vi "Wellington1.vi"() -> ()   [LabVIEW 2009]
uses:
  <vilib>/NXT/Block Support/NXT_InputPort.ctl
  <vilib>/NXT/Block Support/NXT_ButtonSelector.ctl
  <vilib>/NXT/Subs/MotorOutput.ctl
  <vilib>/NXT/Dual Mode Library/Waits/Wait_Num.vi
  <vilib>/NXT/Dual Mode Library/Display/drawText.vi
  <vilib>/NXT/Dual Mode Library/Sensors/Light_On.vi
  <vilib>/NXT/Dual Mode Library/Sensors/Touch_Pressed.vi
  <vilib>/NXT/Dual Mode Library/Sensors/Sound_dB.vi
  <vilib>/NXT/Dual Mode Library/Sensors/Sonar_cm.vi
  <vilib>/NXT/Dual Mode Library/Sensors/readNXTButton.vi
  <vilib>/NXT/Subs/NXT_SteeringOutputPort.ctl
panel:
  out "Cor inicial":i16
  out "Verificacao":bool[](array[boolean])
  out "Toque":bool
  out "Visor":string
  out "Ruído":i16(slide) scale=0.0..100.0
  out "Luminosidade":i16
  out "Distância":i16
  out "Botao":bool
  # "O Mindstorms irá ficar no seguinte loop até que o botão central seja precionado:\nAciona os motores B e C para frente.\nMostrará os valores dos sensores na tela.\nCaso seja detectado: uma distância menor que 50cm, ou um ruído maior que 70dB, ou o sensor de toque seja precionado ou haja uma mudança de cor. O Mindstorms irá executar a seguinte rotina:\nIrá desligar os motores B e C.\nIrá ligar os motores B e C para trás e dará cinco voltas.\nSelecionará aleatoriamente um lado (direita/esquerda).\nEmitirá um som \"äleatório\".\nVirará 180 graus para o lado escolhido.\nE voltará ao loop."
  # "Configuração:\nOUT_A: GARRA\nOUT_B: RODA DA ESQUERDA\nOUT_C: RODA DA DIREITA\nIN_1: SENSOR DE TOQUE\nIN_2: SENSOR SONORO\nIN_3: SENSOR LUMINOSO\nIN_4: SENSOR ULTRA-SOM"
  # "1 - Distância menor que 50cm\n2 - Mudança de cor detectada\n3 - Ruído maior que 70dB\n4 - Toque precionado"
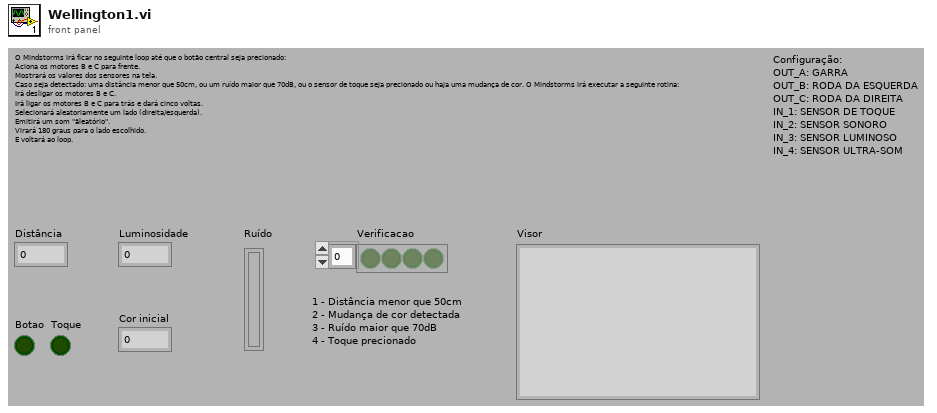
[diagram p1: front panel]
types:
  T1 = typedef "MotorOutput.ctl" = u8
  T2 = typedef "NXT_InputPort.ctl" = u8
  T3 = typedef "LVHSConnector.ctl" = cluster{"error":errorcluster, "address":string, "NXT #":i32, "Show Error":bool, "Connection":u16}
  T4 = typedef "NXT_SteeringOutputPort.ctl" = u16
  T5 = typedef "NXT_ButtonSelector.ctl" = u16
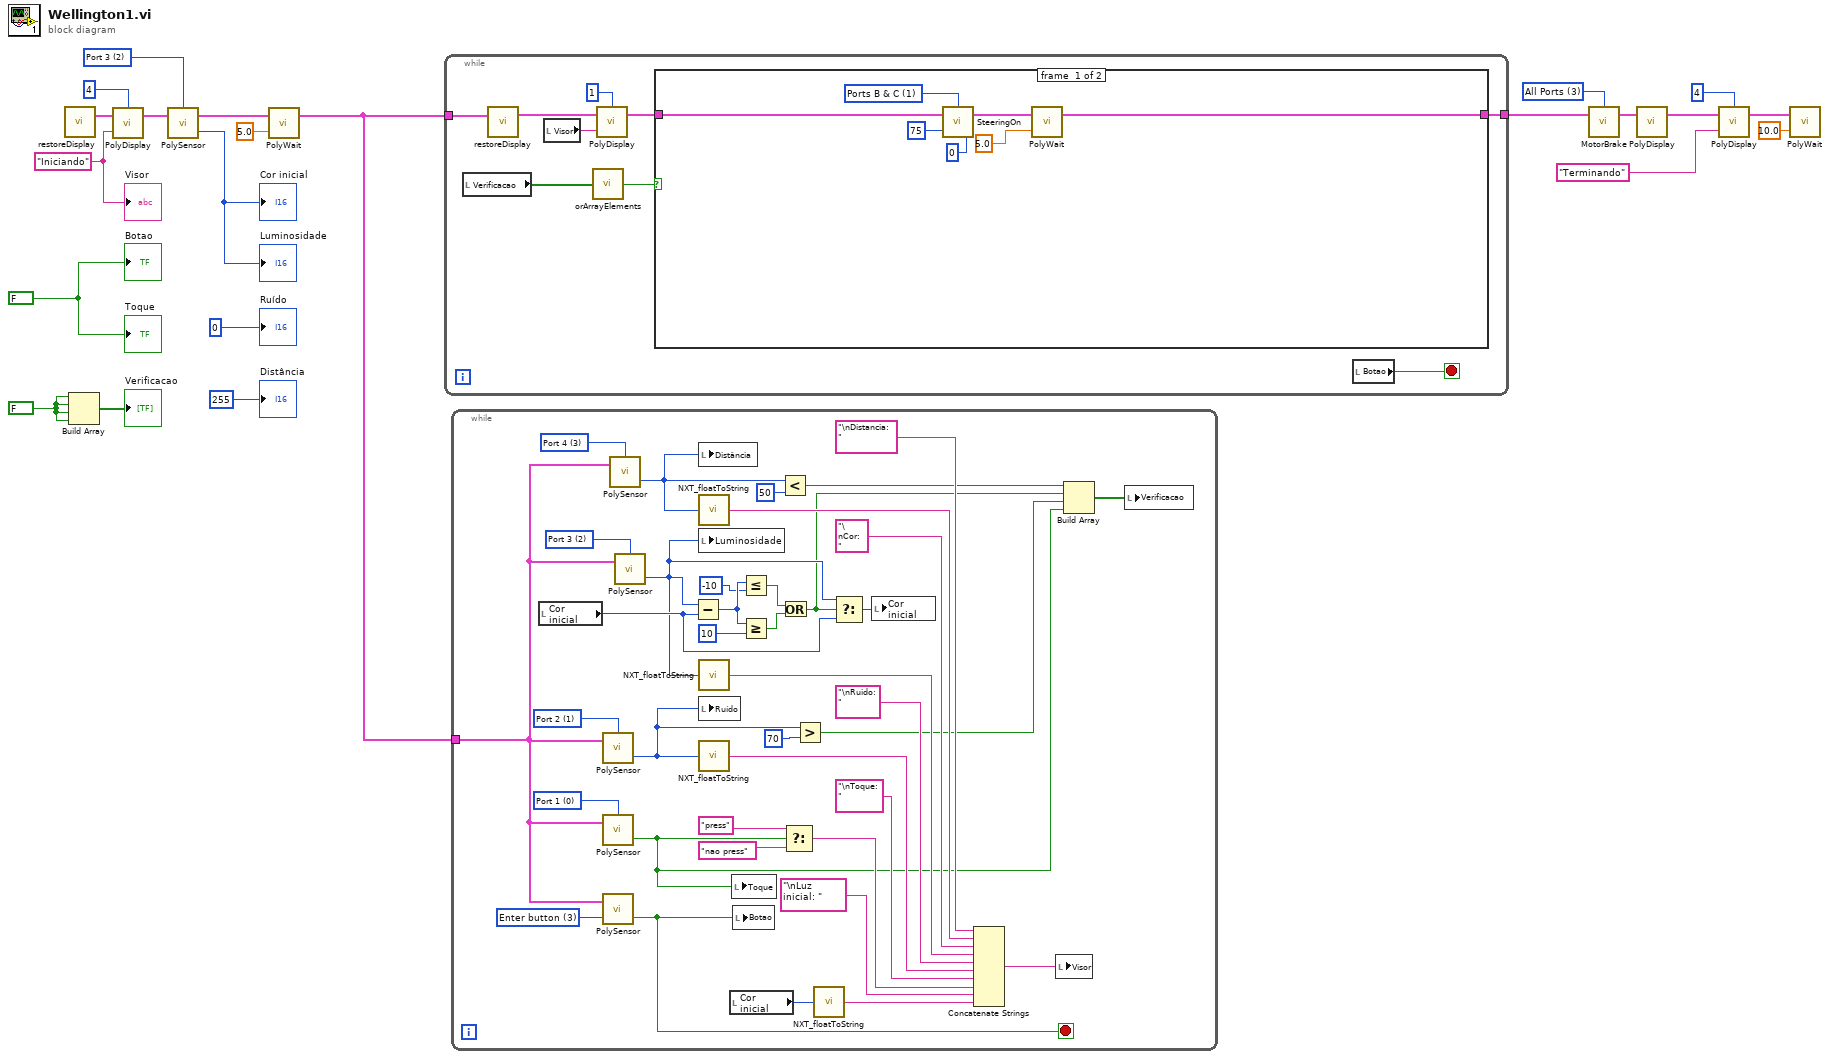
[diagram p0: block diagram]
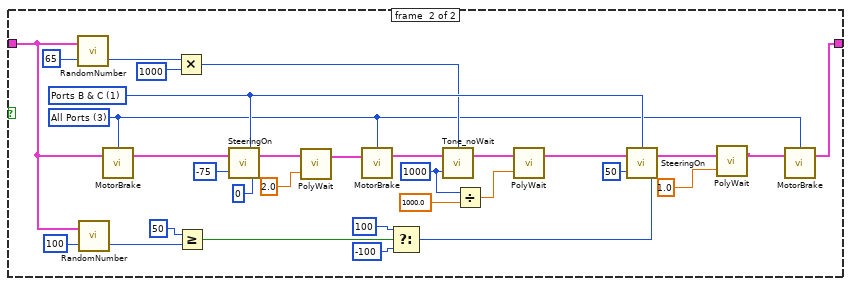
[diagram p2: hidden frame]
diagram:
  w3 = FALSE
  w14 = T1 3 items=["Port A", "Port B", "Port C", "All Ports"] ("Output Port (All Ports)")
  w10 = T2 2 items=["Port 1", "Port 2", "Port 3", "Port 4"] ("Input Port")
  w21 = "Iniciando"
  w20 = FALSE
  n1 = call <vilib>:"restoreDisplay.vi"() -> ("NXT"=w15:T3)  [unwired: 4 in]
  n2 = Build Array(w3, w3, w3, w3) -> (→"Verificacao":bool[])
  n3 = call-poly <vilib>:"PolyDisplay.vi"("Text"=w21, "NXT"=w15, "Line"=i16 4) -> ("NXT"=w7:T3)  [unwired: 1 in]
  n4 = call-poly <vilib>:"PolySensor.vi"("NXT"=w7, "Port (Port 3)"=w10) -> ("Scaled Value"=→"Luminosidade" →"Cor inicial":i16, "NXT"=w8:T3)  [unwired: 1 in]
  n5 = call-poly <vilib>:"PolyWait.vi"("Time (1 sec)"=sgl 5.0, "NXT"=w8) -> ("NXT"=w2:T3)  [unwired: 2 in]
  n6 = while {
    tunnel: w2 -> [w27]
    tunnel: [w23] -> w5
    stop <- w31 stop-if-true
    n7 = local read "Verificacao"() -> (w26:bool[])
    n8 = call <vilib>:"restoreDisplay.vi"("NXT"=w27) -> ("NXT"=w30:T3)  [unwired: 3 in]
    n9 = local read "Visor"() -> (w28:string)
    n10 = call <vilib>:"orArrayElements.vi"("Boolean Array"=w26) -> ("Logical OR"=w24:bool)
    n11 = call-poly <vilib>:"PolyDisplay.vi"("Text"=w28, "NXT"=w30, "Line"=i16 1) -> ("NXT"=w25:T3)  [unwired: 1 in]
    n12 = case shown="False" w24 {
      tunnel: w25 -> [w35 w66]
      tunnel: [w32 w41] -> w23
      frame #0 {
        w36 = T4 1 items=["Ports A & B", "Ports B & C", "Ports A & C"] ("Output Port")
        n13 = call <vilib>:"SteeringOn.vi"("Power (75)"=75, "Steering (100)"=0, "NXT"=w35, "Output Ports"=w36) -> ("NXT"=w34:T3)
        n14 = call-poly <vilib>:"PolyWait.vi"("Time (1 sec)"=sgl 5.0, "NXT"=w34) -> ("NXT"=w32:T3)  [unwired: 2 in]
      }
      frame #1 {
        w50 = u16 1000
        w48 = T1 3 items=["Port A", "Port B", "Port C", "All Ports"] ("Output Port (All Ports)")
        w65 = T4 1 items=["Ports A & B", "Ports B & C", "Ports A & C"] ("Output Port")
        n15 = call <vilib>:"RandomNumber.vi"("Max Value"=i16 65, "NXT"=w66) -> ("Random Number"=w61:u16)  [unwired: 1 in, 1 out]
        n16 = call <vilib>:"RandomNumber.vi"("Max Value"=i16 100, "NXT"=w66) -> ("Random Number"=w57:u16)  [unwired: 1 in, 1 out]
        n17 = call <vilib>:"MotorBrake.vi"("NXT"=w66, "Port (All Ports)"=w48) -> ("NXT"=w40:T3)  [unwired: 2 in]
        n18 = Multiply(x=w61, y=i16 1000) -> (x*y=w59:u16)
        n19 = Greater Or Equal?(x=i16 50, y=w57) -> (x >= y?=w56:bool)
        n20 = call <vilib>:"SteeringOn.vi"("Power (75)"=-75, "Steering (100)"=0, "NXT"=w40, "Output Ports"=w65) -> ("NXT"=w44:T3)
        n21 = call-poly <vilib>:"PolyWait.vi"("Time (1 sec)"=sgl 2.0, "NXT"=w44) -> ("NXT"=w45:T3)  [unwired: 2 in]
        n22 = call <vilib>:"MotorBrake.vi"("NXT"=w45, "Port (All Ports)"=w48) -> ("NXT"=w49:T3)  [unwired: 2 in]
        n23 = Select(t=100, s=w56, f=-100) -> (s? t:f=w58:i32)
        n24 = call <vilib>:"Tone_noWait.vi"("Duration (500 ms)"=w50, "NXT"=w49, "Tone (440 Hz)"=w59) -> ("NXT"=w63:T3)  [unwired: 1 in]
        n25 = Divide(x=w50, y=sgl 1000.0) -> (x/y=w52:sgl)
        n26 = call-poly <vilib>:"PolyWait.vi"("Time (1 sec)"=w52, "NXT"=w63) -> ("NXT"=w39:T3)  [unwired: 2 in]
        n27 = call <vilib>:"SteeringOn.vi"("Power (75)"=50, "Steering (100)"=w58, "NXT"=w39, "Output Ports"=w65) -> ("NXT"=w47:T3)
        n28 = call-poly <vilib>:"PolyWait.vi"("Time (1 sec)"=sgl 1.0, "NXT"=w47) -> ("NXT"=w46:T3)  [unwired: 2 in]
        n29 = call <vilib>:"MotorBrake.vi"("NXT"=w46, "Port (All Ports)"=w48) -> ("NXT"=w41:T3)  [unwired: 2 in]
      }
    }
    n30 = local read "Botao"() -> (w31:bool)
  }
  n31 = while {
    tunnel: w2 -> [w72]
    stop <- w71 stop-if-true
    w92 = T5 3 items=["Enter button"=3, "Left button"=2, "Right button"=1] ("Button (Enter button)")
    w104 = T2 3 items=["Port 1", "Port 2", "Port 3", "Port 4"] ("Input Port")
    w105 = T2 2 items=["Port 1", "Port 2", "Port 3", "Port 4"] ("Input Port")
    w106 = T2 1 items=["Port 1", "Port 2", "Port 3", "Port 4"] ("Input Port")
    w107 = T2 0 items=["Port 1", "Port 2", "Port 3", "Port 4"] ("Input Port")
    n32 = local read "Cor inicial"() -> (w81:i16)
    n33 = call-poly <vilib>:"PolySensor.vi"("NXT"=w72, "Port (Port 2)"=w106) -> ("Sound (dB)"=w77:i16)  [unwired: 1 in, 1 out]
    n34 = call-poly <vilib>:"PolySensor.vi"("NXT"=w72, "Port (Port 1)"=w107) -> ("Yes / No"=w70:bool)  [unwired: 1 in, 1 out]
    n35 = call-poly <vilib>:"PolySensor.vi"("Button (Enter button)"=w92, "NXT"=w72) -> ("Yes/No"=w71:bool)  [unwired: 1 in, 1 out]
    n36 = call-poly <vilib>:"PolySensor.vi"("NXT"=w72, "Port (Port 4)"=w104) -> ("Distance (cm)"=w88:i16)  [unwired: 1 in, 1 out]
    n37 = call-poly <vilib>:"PolySensor.vi"("NXT"=w72, "Port (Port 3)"=w105) -> ("Scaled Value"=w80:i16)  [unwired: 1 in, 1 out]
    n38 = Subtract(x=w80, y=w81) -> (x-y=w74:i16)
    n39 = local write "Distância"(w88) -> ()
    n40 = call <vilib>:"NXT_floatToString.vi"("number"=w88) -> ("string"=w100:string)
    n41 = local write "Luminosidade"(w80) -> ()
    n42 = call <vilib>:"NXT_floatToString.vi"("number"=w80) -> ("string"=w98:string)
    n43 = local write "Ruído"(w77) -> ()
    n44 = call <vilib>:"NXT_floatToString.vi"("number"=w77) -> ("string"=w95:string)
    n45 = local read "Cor inicial"() -> (w91:i16)
    n46 = local write "Toque"(w70) -> ()
    n47 = local write "Botao"(w71) -> ()
    n48 = Less Or Equal?(x=w74, y=i16 -10) -> (x <= y?=w82:bool)
    n49 = Greater Or Equal?(x=w74, y=i16 10) -> (x >= y?=w83:bool)
    n50 = Less?(x=w88, y=i16 50) -> (x < y?=w86:bool)
    n51 = Or(x=w82, y=w83) -> (x .or. y?=w79:bool)
    n52 = Select(t="press", s=w70, f="nao press") -> (s? t:f=w96:string)
    n53 = Greater?(x=w77, y=i16 70) -> (0:w76:bool)
    n54 = call <vilib>:"NXT_floatToString.vi"("number"=w91) -> ("string"=w89:string)
    n55 = Select(t=w80, s=w79, f=w81) -> (s? t:f=w85:i16)
    n56 = local write "Cor inicial"(w85) -> ()
    n57 = Concatenate Strings("\nDistancia: ", w100, "\nCor: ", w98, "\nRuido: ", w95, "\nToque: ", w96, "\nLuz inicial: ", w89) -> (w93:string)
    n58 = local write "Visor"(w93) -> ()
    n59 = Build Array(w86, w79, w76, w70) -> (w75:bool[])
    n60 = local write "Verificacao"(w75) -> ()
  }
  n61 = call <vilib>:"MotorBrake.vi"("NXT"=w5, "Port (All Ports)"=w14) -> ("NXT"=w12:T3)  [unwired: 2 in]
  n62 = call-poly <vilib>:"PolyDisplay.vi"("NXT"=w12) -> ("NXT"=w18:T3)  [unwired: 3 in]
  n63 = call-poly <vilib>:"PolyDisplay.vi"("Text"="Terminando", "NXT"=w18, "Line"=i16 4) -> ("NXT"=w11:T3)  [unwired: 1 in]
  n64 = call-poly <vilib>:"PolyWait.vi"("Time (1 sec)"=sgl 10.0, "NXT"=w11) -> ()  [unwired: 2 in, 1 out]
  "Botao" <- w20
  "Distância" <- i16 255
  "Ruído" <- i16 0
  "Visor" <- w21
  "Toque" <- w20
